vi "Close.vi"(8 "error in (no error)":errorcluster, 11 "TcpSocket in":refnum<class "TcpSocket.lvclass">) -> (0 "error out":errorcluster, 3 "TcpSocket out":refnum<class "TcpSocket.lvclass">)   [LabVIEW 2021, in "TcpSocket.lvlib" / "TcpSocket.lvclass"]
uses:
  TcpSocket.lvclass
  TcpSocket.lvclass/TcpSocket.ctl
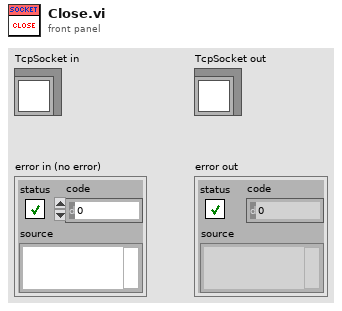
[diagram p1: front panel]
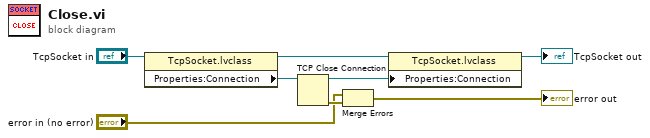
[diagram p0: block diagram]
diagram:
  n1 = property class="TcpSocket.lvclass"(reference="TcpSocket in") -> (reference out=w7:refnum<class "TcpSocket.lvclass">, "Properties:Connection"=w6:refnum<k5>)  [unwired: 1 in, 1 out]
  n2 = TCP Close Connection(connection ID=w6) -> (connection ID out=w5:refnum<k5>, error out=w8:errorcluster)  [unwired: 2 in]
  n3 = Merge Errors("error in (no error)", w8) -> (→"error out":errorcluster)
  n4 = property class="TcpSocket.lvclass"(reference=w7, "Properties:Connection"=w5) -> (reference out=→"TcpSocket out":refnum<class "TcpSocket.lvclass">)  [unwired: 1 in, 1 out]
